vi "Barcode.vi"(9 "流水号":string, 10 "年月日":string, 11 "start (0, 0)":cluster{"start row":i32, "start column":i32}={"start row"=1, "start column"=1}) -> (3 "条形码":string)   [LabVIEW 2020]
uses:
  Sources/Global_Variable/Global.vi
panel:
  out "结果字符串":string
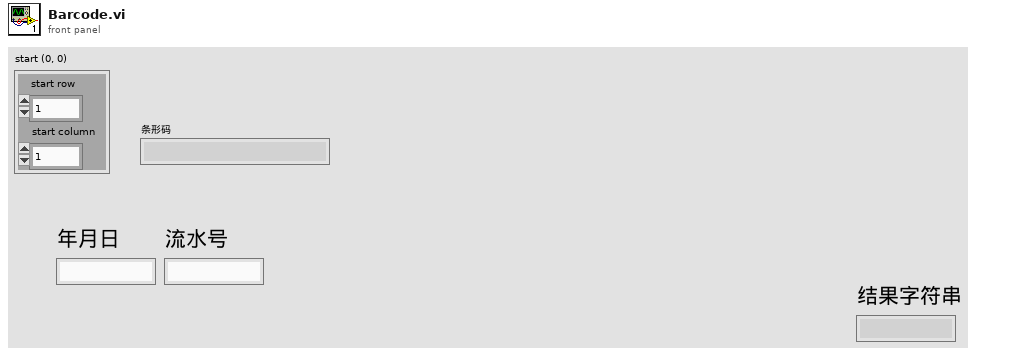
[diagram p1: front panel]
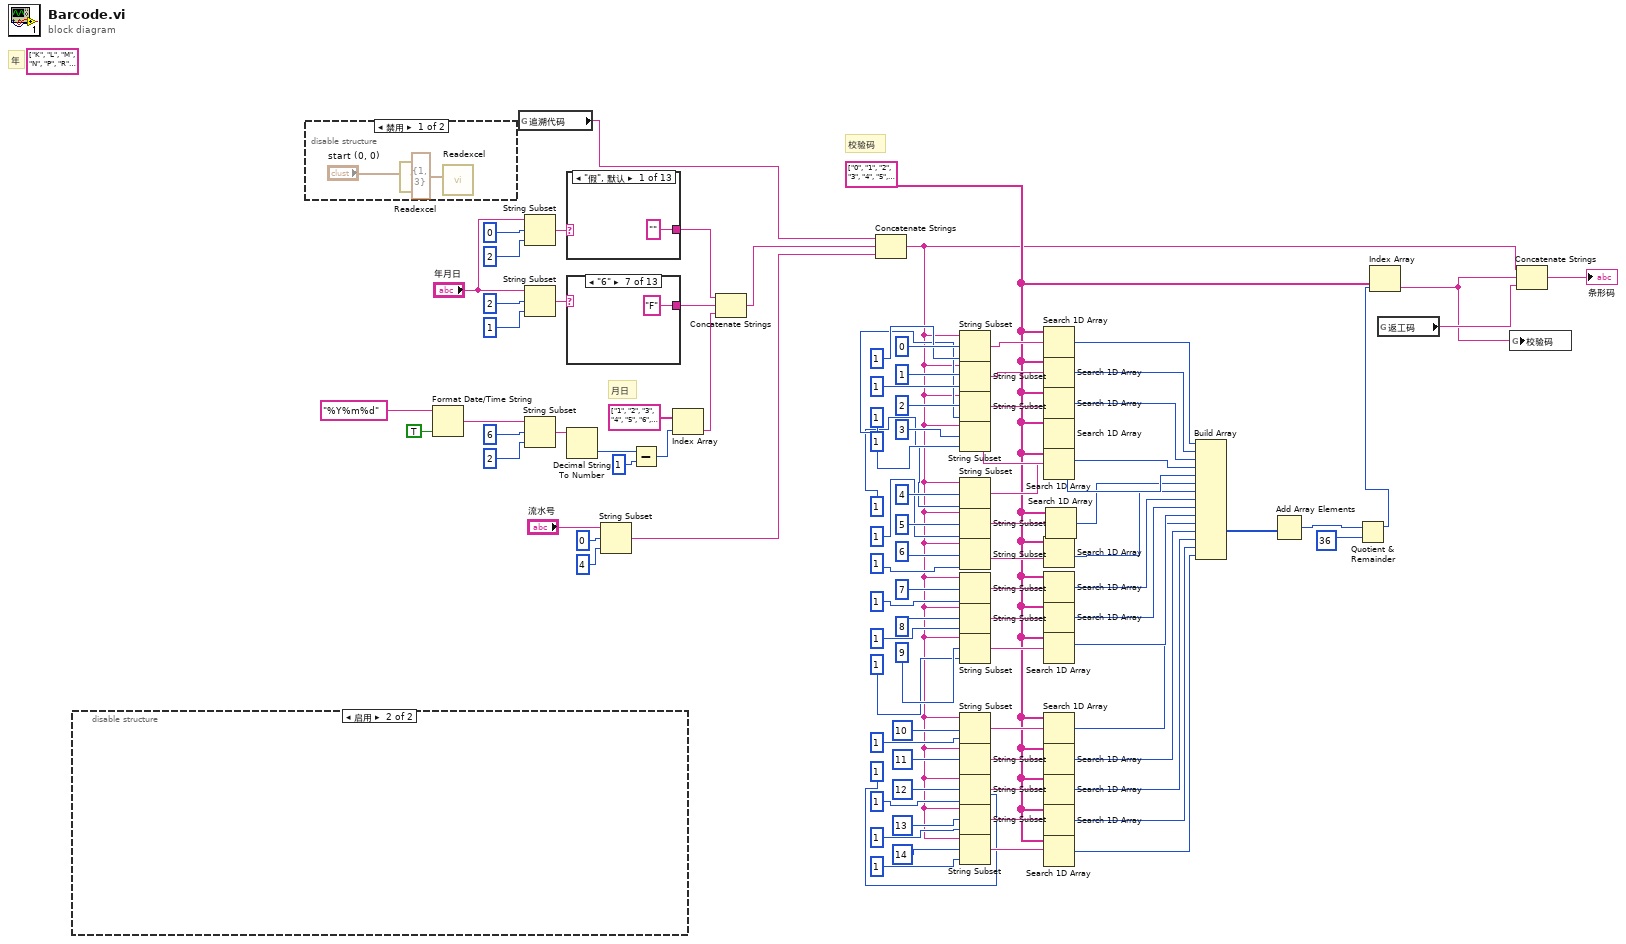
[diagram p0: block diagram]
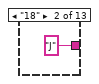
[diagram p3: hidden frame]
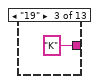
[diagram p4: hidden frame]
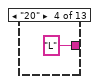
[diagram p5: hidden frame]
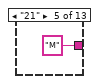
[diagram p6: hidden frame]
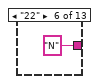
[diagram p7: hidden frame]
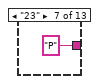
[diagram p8: hidden frame]
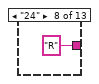
[diagram p9: hidden frame]
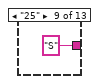
[diagram p10: hidden frame]
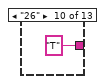
[diagram p11: hidden frame]
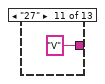
[diagram p12: hidden frame]
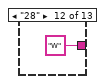
[diagram p13: hidden frame]
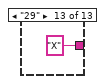
[diagram p14: hidden frame]
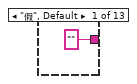
[diagram p15: hidden frame]
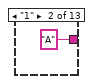
[diagram p16: hidden frame]
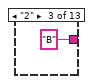
[diagram p17: hidden frame]
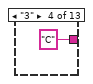
[diagram p18: hidden frame]
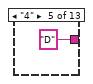
[diagram p19: hidden frame]
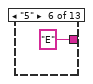
[diagram p20: hidden frame]
diagram:
  w19 = string[] ["0", "1", "2", "3", "4", "5", "6", "7", "8", "9", "A", "B", "C", "D", "E", "F", "G", "H", "I", "J", "K", "L", "M", "N", "O", "P", "Q", "R", "S", "T", "U", "V", "W", "X", "Y", "Z"]
  (unwired) string[] ["K", "L", "M", "N", "P", "R", "S", "T", "V", "W", "X", "Y", "0"]
  # "校验码"
  # "月日"
  # "年"
  n1 = disable-structure shown="启用" {
    frame Disabled {
      n2 = call <vilib>:"Application Directory.vi"() -> ("Application Directory"=w103:path)
      n3 = Build Path(base path=w103, name or relative path="流水号配置.ini" ("名称或相对路径")) -> (appended path=w101:path)
      n4 = call "写配置.vi"("配置文件路径"=w101, "枚举"=enum16{"写", "读"}."读", "section"="R128,R527,R538,R92") -> ("读取值"=w100:u32)  [unwired: 8 in]
      n5 = Decrement(x=w100) -> (x-1=w99:u32)
      n6 = Add(x=u32 1, y=w99) -> (x+y=w107:u32)
      n7 = Quotient & Remainder(x=w107, y=u32 1000) -> (x-y*floor(x/y)=w98:u32)  [unwired: 1 out]
      n8 = Format Into String(format string="%04d" ("格式字符串"), w98) -> (resulting string=→"结果字符串":string)  [unwired: 2 in, 1 out]
      n9 = Increment(x=w98) -> (x+1=w97:u32)
      n10 = call "写配置.vi"("配置文件路径"=w101, "枚举"=enum16{"写", "读"}."写", "section"="R128,R527,R538,R92", "写入值"=w97) -> ()  [unwired: 7 in, 1 out]
    }
    frame Enabled {
    }
  }
  n11 = disable-structure shown="禁用" {
    frame Disabled {
      n12 = call "Readexcel.vi"("start (0, 0)"="start (0, 0)") -> ()  [unwired: 10 in, 1 out]
      n13 = call "Readexcel.vi"("start (0, 0)"=cluster{"start row":i32, "start column":i32} {"start row"=1, "start column"=3}) -> ()  [unwired: 10 in, 1 out]
    }
    frame Enabled {
    }
  }
  n14 = Format Date/Time String(time format string (%c)="%Y%m%d" ("时间格式字符串(%c)"), UTC format=TRUE ("UTC格式")) -> (date/time string=w11:string)  [unwired: 1 in]
  n15 = global read "Global.vi" "追溯代码"() -> (w3:string)
  n16 = String Subset(string="年月日", offset (0)=0 ("偏移量(0)"), length (rest)=2 ("长度（剩余）")) -> (substring=w5:string)
  n17 = String Subset(string="年月日", offset (0)=2 ("偏移量(0)"), length (rest)=1 ("长度（剩余）")) -> (substring=w6:string)
  n18 = String Subset(string=w11, offset (0)=6 ("偏移量(0)"), length (rest)=2 ("长度（剩余）")) -> (substring=w88:string)
  n19 = case shown="\"假\", 默认" w5 {
    tunnel: ["" "J" "K" "L" "M" "N" "P" "R" "S" "T" "V" "W" "X"] -> w4
    frame "假", Default {
    }
    frame "18" {
    }
    frame "19" {
    }
    frame "20" {
    }
    frame "21" {
    }
    frame "22" {
    }
    frame "23" {
    }
    frame "24" {
    }
    frame "25" {
    }
    frame "26" {
    }
    frame "27" {
    }
    frame "28" {
    }
    frame "29" {
    }
  }
  n20 = case shown="\"6\"" w6 {
    tunnel: ["" "A" "B" "C" "D" "E" "F" "G" "H" "J" "K" "L" "M"] -> w10
    frame "假", Default {
    }
    frame "1" {
    }
    frame "2" {
    }
    frame "3" {
    }
    frame "4" {
    }
    frame "5" {
    }
    frame "6" {
    }
    frame "7" {
    }
    frame "8" {
    }
    frame "9" {
    }
    frame "A" {
    }
    frame "B" {
    }
    frame "C" {
    }
  }
  n21 = Decimal String To Number(string=w88) -> (number=w23:i32)  [unwired: 2 in, 1 out]
  n22 = String Subset(string="流水号", offset (0)=0 ("偏移量(0)"), length (rest)=4 ("长度（剩余）")) -> (substring=w14:string)
  n23 = Subtract(x=w23, y=1) -> (x-y=w24:i32)
  n24 = Index Array(array=string[] ["1", "2", "3", "4", "5", "6", "7", "8", "9", "A", "B", "C", "D", "E", "F", "G", "H", "J", "K", "L", "M", "N", "P", "R", "S", "T", "U", "V", "W", "X", "Y", "0"], index=w24) -> (element=w87:string)
  n25 = Concatenate Strings(w4, w10, w87) -> (w21:string)
  n26 = Concatenate Strings(w3, w21, w14) -> (w17:string)
  n27 = String Subset(string=w17, offset (0)=0 ("偏移量(0)"), length (rest)=1 ("长度（剩余）")) -> (substring=w86:string)
  n28 = String Subset(string=w17, offset (0)=1 ("偏移量(0)"), length (rest)=1 ("长度（剩余）")) -> (substring=w82:string)
  n29 = String Subset(string=w17, offset (0)=2 ("偏移量(0)"), length (rest)=1 ("长度（剩余）")) -> (substring=w81:string)
  n30 = String Subset(string=w17, offset (0)=3 ("偏移量(0)"), length (rest)=1 ("长度（剩余）")) -> (substring=w80:string)
  n31 = String Subset(string=w17, offset (0)=4 ("偏移量(0)"), length (rest)=1 ("长度（剩余）")) -> (substring=w79:string)
  n32 = String Subset(string=w17, offset (0)=5 ("偏移量(0)"), length (rest)=1 ("长度（剩余）")) -> (substring=w78:string)
  n33 = String Subset(string=w17, offset (0)=6 ("偏移量(0)"), length (rest)=1 ("长度（剩余）")) -> (substring=w77:string)
  n34 = String Subset(string=w17, offset (0)=7 ("偏移量(0)"), length (rest)=1 ("长度（剩余）")) -> (substring=w76:string)
  n35 = String Subset(string=w17, offset (0)=8 ("偏移量(0)"), length (rest)=1 ("长度（剩余）")) -> (substring=w75:string)
  n36 = String Subset(string=w17, offset (0)=9 ("偏移量(0)"), length (rest)=1 ("长度（剩余）")) -> (substring=w74:string)
  n37 = String Subset(string=w17, offset (0)=10 ("偏移量(0)"), length (rest)=1 ("长度（剩余）")) -> (substring=w73:string)
  n38 = String Subset(string=w17, offset (0)=11 ("偏移量(0)"), length (rest)=1 ("长度（剩余）")) -> (substring=w72:string)
  n39 = String Subset(string=w17, offset (0)=12 ("偏移量(0)"), length (rest)=1 ("长度（剩余）")) -> (substring=w71:string)
  n40 = String Subset(string=w17, offset (0)=13 ("偏移量(0)"), length (rest)=1 ("长度（剩余）")) -> (substring=w70:string)
  n41 = String Subset(string=w17, offset (0)=14 ("偏移量(0)"), length (rest)=1 ("长度（剩余）")) -> (substring=w69:string)
  n42 = Search 1D Array(1D array=w19, element=w86) -> (index of element=w68:i32)  [unwired: 1 in]
  n43 = Search 1D Array(1D array=w19, element=w82) -> (index of element=w67:i32)  [unwired: 1 in]
  n44 = Search 1D Array(1D array=w19, element=w81) -> (index of element=w66:i32)  [unwired: 1 in]
  n45 = Search 1D Array(1D array=w19, element=w80) -> (index of element=w65:i32)  [unwired: 1 in]
  n46 = Search 1D Array(1D array=w19, element=w79) -> (index of element=w64:i32)  [unwired: 1 in]
  n47 = Search 1D Array(1D array=w19, element=w77) -> (index of element=w20:i32)  [unwired: 1 in]
  n48 = Search 1D Array(1D array=w19, element=w76) -> (index of element=w63:i32)  [unwired: 1 in]
  n49 = Search 1D Array(1D array=w19, element=w75) -> (index of element=w62:i32)  [unwired: 1 in]
  n50 = Search 1D Array(1D array=w19, element=w74) -> (index of element=w61:i32)  [unwired: 1 in]
  n51 = Search 1D Array(1D array=w19, element=w73) -> (index of element=w60:i32)  [unwired: 1 in]
  n52 = Search 1D Array(1D array=w19, element=w72) -> (index of element=w59:i32)  [unwired: 1 in]
  n53 = Search 1D Array(1D array=w19, element=w71) -> (index of element=w58:i32)  [unwired: 1 in]
  n54 = Search 1D Array(1D array=w19, element=w70) -> (index of element=w57:i32)  [unwired: 1 in]
  n55 = Search 1D Array(1D array=w19, element=w69) -> (index of element=w56:i32)  [unwired: 1 in]
  n56 = Search 1D Array(1D array=w19, element=w78) -> (index of element=w16:i32)  [unwired: 1 in]
  n57 = Build Array(w68, w67, w66, w65, w64, w16, w20, w63, w62, w61, w60, w59, w58, w57, w56) -> (w55:i32[])
  n58 = Add Array Elements(numeric array=w55) -> (sum=w54:i32)
  n59 = Quotient & Remainder(x=w54, y=36) -> (x-y*floor(x/y)=w18:i32)  [unwired: 1 out]
  n60 = Index Array(array=w19, index=w18) -> (element=w1:string)
  n61 = global read "Global.vi" "返工码"() -> (w2:string)
  n62 = global write "Global.vi" "校验码"(w1) -> ()
  n63 = Concatenate Strings(w17, w1, w2) -> (→"条形码":string)
